vi "RS_SMBV100A_ASKCONFIGURATION.vi"(0 "DriverConnect in":T2={"InterfaceType"=enum."VISA", "OpenedSession"="", "InterfaceSettings"={"Interface"=enum."RS232", "EOS 4 read"=enum."LF (\\n)", "EOS 4 write"=enum."LF (\\n)", "TMO, ms"=10000, "Sett"=variant(cluster{"Baud Rate":u32, "Data Bits":u16, "Parity":u16, "Stop Bits":u16, "Flow Control":u16, "Eho":bool} {"Baud Rate"=75, "Data Bits"=0, "Parity"=0, "Stop Bits"=0, "Flow Control"=0, "Eho"=FALSE})}}, 1 "BASEBAND":string, 9 "Error In":errorcluster) -> (4 "DriverConnect out":T2={"InterfaceType"=enum."VISA", "OpenedSession"="", "InterfaceSettings"={"Interface"=enum."RS232", "EOS 4 read"=enum."LF (\\n)", "EOS 4 write"=enum."LF (\\n)", "TMO, ms"=10000, "Sett"=variant(cluster{"Baud Rate":u32, "Data Bits":u16, "Parity":u16, "Stop Bits":u16, "Flow Control":u16, "Eho":bool} {"Baud Rate"=75, "Data Bits"=0, "Parity"=0, "Stop Bits"=0, "Flow Control"=0, "Eho"=FALSE})}}, 6 "Parsing Satelite":T1, 10 "Error Out":errorcluster)   [LabVIEW 2018]
uses:
  MOKO_LabViewLibrary/MokoLowLevel/MokoLowLovelControl/MLLC_ConnectCluster.ctl
  MOKO_LabViewLibrary/MokoLowLevel/MokoLowLovelControl/MLLC_InterfaceType.ctl
  MOKO_LabViewLibrary/MokoLowLevel/MokoLowLovelControl/MLLC_OpenedSession.ctl
  MOKO_LabViewLibrary/MokoLowLevel/MokoLowLovelControl/MLLC_InterfaceSettings.ctl
  MOKO_LabViewLibrary/MokoLowLevel/MokoLowLovelControl/MLLC_InterfaceKind.ctl
  RS_SMBV100A_Parsing Satelite.ctl
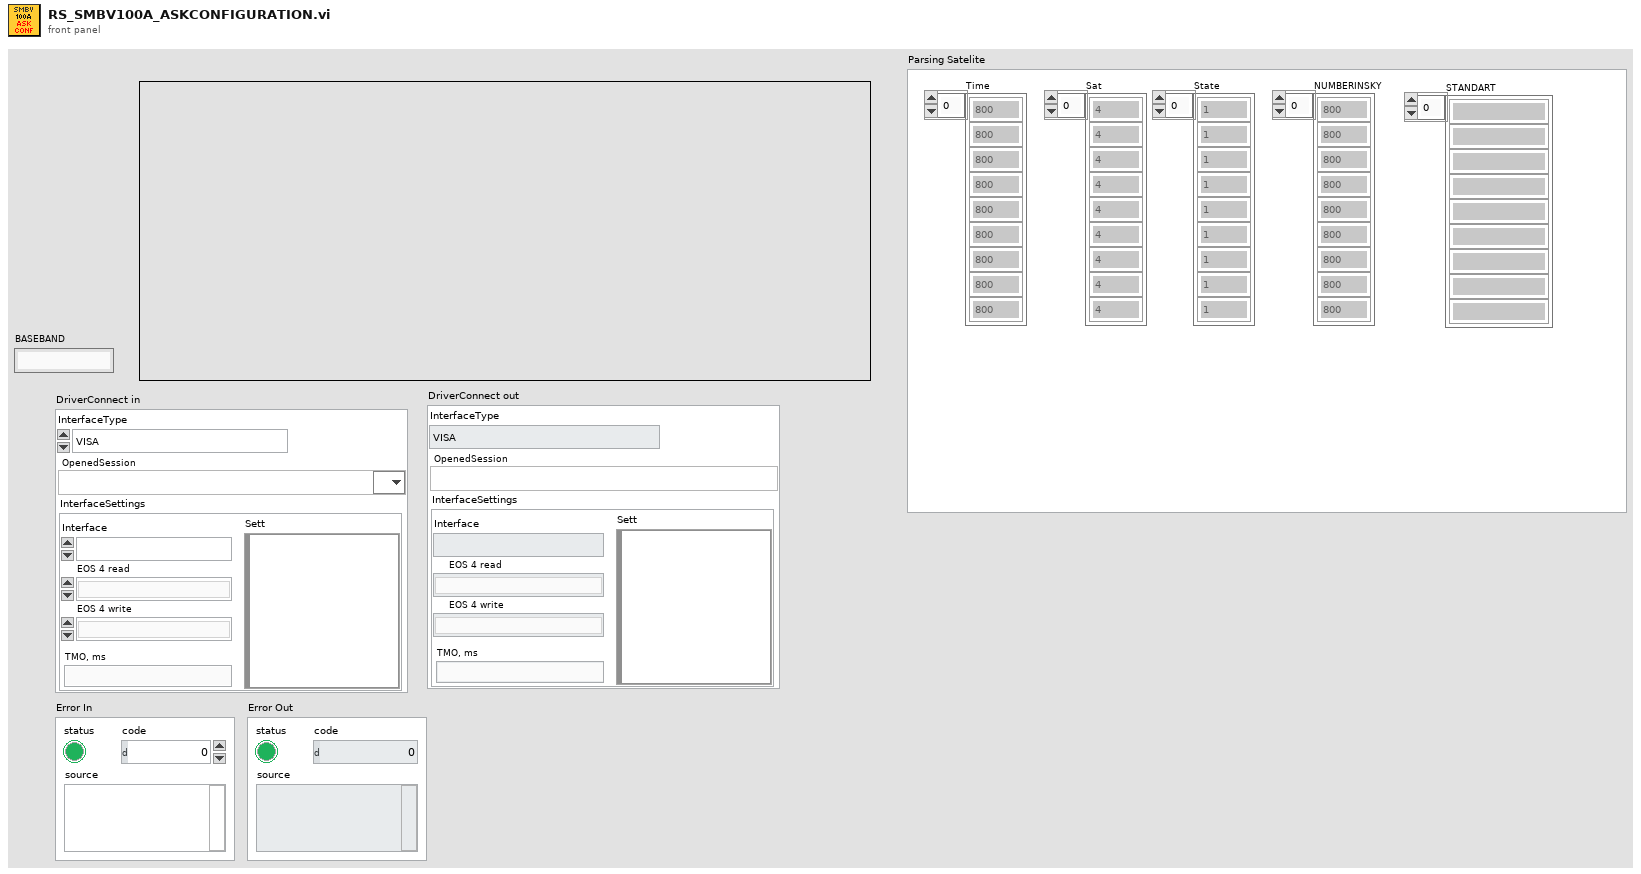
[diagram p1: front panel]
types:
  T1 = typedef "RS_SMBV100A_Parsing Satelite.ctl" = cluster{"Time":dbl[], "Sat":dbl[], "State":dbl[], "NUMBERINSKY":dbl[], "STANDART":string[]}
  T2 = typedef "MLLC_ConnectCluster.ctl" = cluster{"InterfaceType":T3, "OpenedSession":T4, "InterfaceSettings":T5}
  T3 = typedef "MLLC_InterfaceType.ctl" = enum16{"VISA", "Prologix USB-GPIB"}
  T4 = typedef "MLLC_OpenedSession.ctl" = refnum<visa-resource-name>
  T5 = typedef "MLLC_InterfaceSettings.ctl" = cluster{"Interface":T6, "EOS 4 read":enum16{"Default (=EOS 4 write)", "CR (\\r)", "LF (\\n)", "None"}, "EOS 4 write":enum16{"CR+LF (\\r\\n)", "CR (\\r)", "LF (\\n)", "None"}, "TMO, ms":i32, "Sett":variant}
  T6 = typedef "MLLC_InterfaceKind.ctl" = enum16{"RS232", "GPIB", "USB", "Ethernet", "another"}
  T7 = typedef "MLLC_Error.ctl" = errorcluster
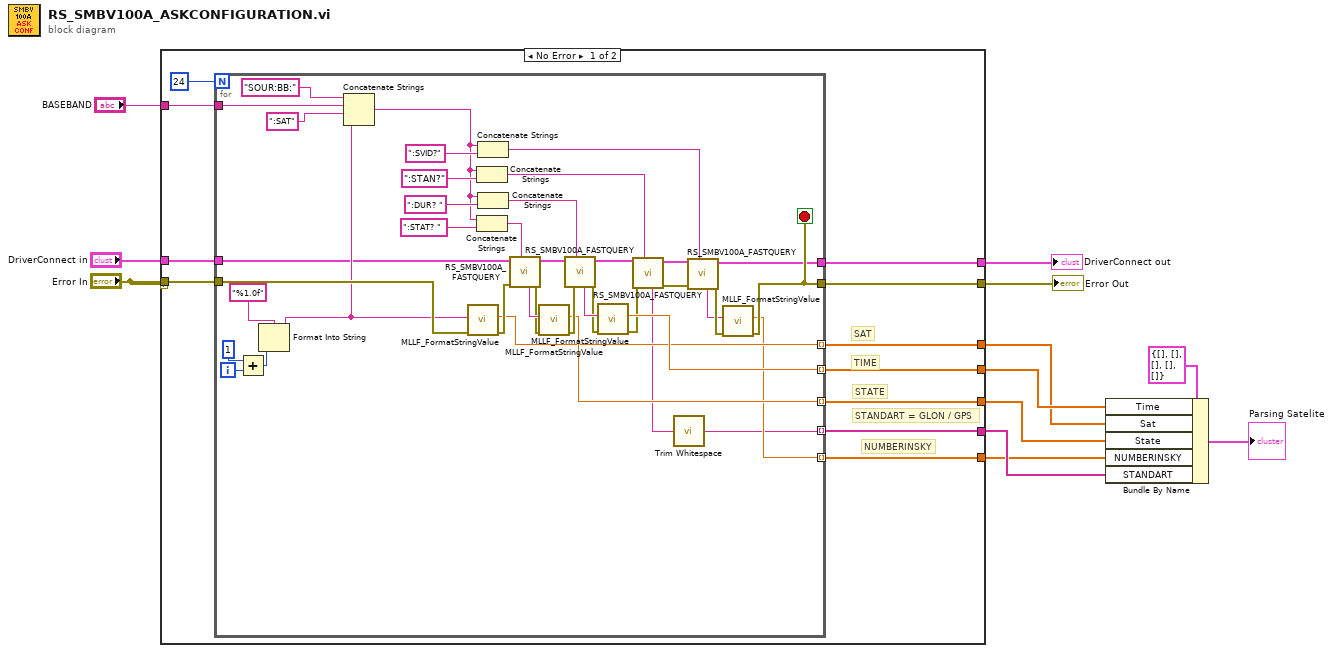
[diagram p0: block diagram]
diagram:
  w6 = T1 {"Time"=[], "Sat"=[], "State"=[], "NUMBERINSKY"=[], "STANDART"=[]} ("Parsing Satelite")
  n1 = case shown="No Error" "Error In" {
    tunnel: "Error In" -> [w21 w64]
    tunnel: "DriverConnect in" -> [w20 w63]
    tunnel: [w19 _] -> w5
    tunnel: [w18 _] -> w4
    tunnel: [w17 _] -> w3
    tunnel: [w16 _] -> w2
    tunnel: [w15 w63] -> w7
    tunnel: [w14 w64] -> w9
    tunnel: [w13 _] -> w1
    tunnel: "BASEBAND" -> [w12 _]
    frame No Error {
      # "NUMBERINSKY"
      # "STANDART = GLON / GPS"
      # "SAT"
      # "STATE"
      # "TIME"
      n2 = for {
        N: 24 -> [_]
        tunnel: w20 -> [w23]
        tunnel: [w47] -> w19 mode=indexing
        tunnel: [w46] -> w17 mode=indexing
        tunnel: [w45] -> w18 mode=indexing
        tunnel: w21 -> [w44]
        tunnel: [w29] -> w16 mode=indexing
        tunnel: [w34] -> w15
        tunnel: [w35] -> w14
        tunnel: [w31] -> w13 mode=indexing
        tunnel: w12 -> [w28]
        i -> [w61]
        stop <- w35 stop-if-true
        n3 = Add(x=1, y=w61) -> (x+y=w57:i32)
        n4 = Format Into String(format string="%1.0f" ("format"), w57) -> (resulting string=w25:string)  [unwired: 2 in, 1 out]
        n5 = Concatenate Strings("SOUR:BB:" ("regular expression"), w28, ":SAT" ("regular expression"), w25) -> (w24:string)
        n6 = call "MLLF_FormatStringValue.vi"("error in"=w44, "String Value"=w25) -> ("error out"=w48:T7, "number"=w45:dbl)  [unwired: 7 in, 1 out]
        n7 = Concatenate Strings(w24, ":STAN?" ("regular expression")) -> (w40:string)
        n8 = Concatenate Strings(w24, ":STAT? " ("regular expression")) -> (w52:string)
        n9 = Concatenate Strings(w24, ":SVID?" ("regular expression")) -> (w33:string)
        n10 = Concatenate Strings(w24, ":DUR? " ("regular expression")) -> (w53:string)
        n11 = call "RS_SMBV100A_FASTQUERY.vi"("input"=w52, "Error In"=w48, "DriverConnect in"=w23) -> ("Error Out"=w50:errorcluster, "DriverConnect out"=w54:T2, "output"=w51:string)  [unwired: 6 in]
        n12 = call "MLLF_FormatStringValue.vi"("error in"=w50, "String Value"=w51) -> ("error out"=w49:T7, "number"=w46:dbl)  [unwired: 7 in, 1 out]
        n13 = call "RS_SMBV100A_FASTQUERY.vi"("input"=w53, "Error In"=w49, "DriverConnect in"=w54) -> ("Error Out"=w59:errorcluster, "DriverConnect out"=w43:T2, "output"=w62:string)  [unwired: 6 in]
        n14 = call "MLLF_FormatStringValue.vi"("error in"=w59, "String Value"=w62) -> ("error out"=w42:T7, "number"=w47:dbl)  [unwired: 7 in, 1 out]
        n15 = call "RS_SMBV100A_FASTQUERY.vi"("input"=w40, "Error In"=w42, "DriverConnect in"=w43) -> ("Error Out"=w36:errorcluster, "DriverConnect out"=w37:T2, "output"=w30:string)  [unwired: 6 in]
        n16 = call <vilib>:"Trim Whitespace.vi"("string"=w30) -> ("trimmed string"=w29:string)  [unwired: 1 in]
        n17 = call "RS_SMBV100A_FASTQUERY.vi"("input"=w33, "Error In"=w36, "DriverConnect in"=w37) -> ("Error Out"=w38:errorcluster, "DriverConnect out"=w34:T2, "output"=w32:string)  [unwired: 6 in]
        n18 = call "MLLF_FormatStringValue.vi"("error in"=w38, "String Value"=w32) -> ("error out"=w35:T7, "number"=w31:dbl)  [unwired: 7 in, 1 out]
      }
    }
    frame Error {
    }
  }
  "Error Out" <- w9
  "DriverConnect out" <- w7
  n19 = Bundle By Name(cluster=w6, "Time"=w5, "Sat"=w4, "State"=w3, "NUMBERINSKY"=w1, "STANDART"=w2) -> ()  [unwired: 1 out]
  "Parsing Satelite" <- w6
